vi "Main.vi"(0 "?":bool, 3 "P_max":dbl, 4 "Numbers_of_\nsamples":i32, 5 "V_max":dbl, 6 "V_min":dbl) -> (1 "Progress":u8(slide) scale=0.0..100.0, 2 "I=f(U)":cluster{dbl[], dbl[]}(graph))   [LabVIEW 2020]
doc: "Main VI with state machine.\nMain functions:\n- Ploting graph in real time (Measurment button),\n- Exporting to MS Excel file (Save button),\n- Emergency stop (Stop button),\n- Shutting down application (Exit button)\nInputs:\n- Minimal voltage,\n- Maximum Voltage,\n- Threshold current,\n- Maximum power,\n- Number of measurement samples,\nVisual representation:\n- Graph,\n- Handsome_meater (light on when handsom graph is ploted),\n- Chadomeater (light on when everything is alright),\n- Progressbar,\nExtra features:\n- Playing music during computing,\n- Showing up Cleopatra at the and of measurments,\n- Shuting down with additional sound and picture."
uses:
  <vilib>/sound2/lvsound2.llb/Sound Output Task ID.ctl
  controls/State.ctl
  <vilib>/Analysis/1siggen.llb/Ramp Pattern by Samples.vi
  <vilib>/Utility/error.llb/Error Cluster From Error Code.vi
  <vilib>/ErrorRing/Error Ring.xnode
  <vilib>/Analysis/NI_AALBase.lvlib
panel:
  out "path":path
  out "task ID 2":T1 format="%.0x"
  out "?":picture
  out "2D Picture":picture
  out "task ID":T1 format="%.0x"
  in  "I_max":dbl
  out "Handsom_meter":bool
  out "Chadometer":bool
  in  "?":bool
  in  "?":bool
  in  "?":bool
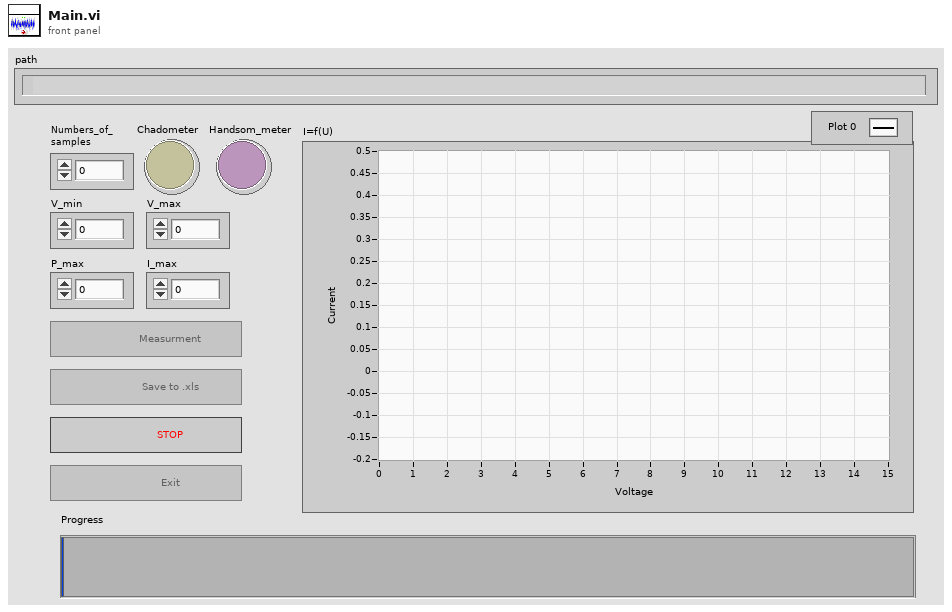
[diagram p1: front panel]
types:
  T1 = typedef "Sound Output Task ID.ctl" = u32
  T2 = typedef "State.ctl" = enum16{"Initialize", "Wait for Event", "Measure", "Save", "Exit"}
  T3 = enum8{"Enabled", "Disabled", "Disabled and Grayed Out"}
  T4 = typedef "imagedata.ctl" = cluster{"image type":i32, "image depth":i32, "image":u8[], "mask":u8[], "colors":u32[], "Rectangle":cluster{"left":i16, "top":i16, "right":i16, "bottom":i16}}
  T5 = typedef "LVBoundsTypeDef.ctl" = cluster{"Width":u32, "Height":u32}
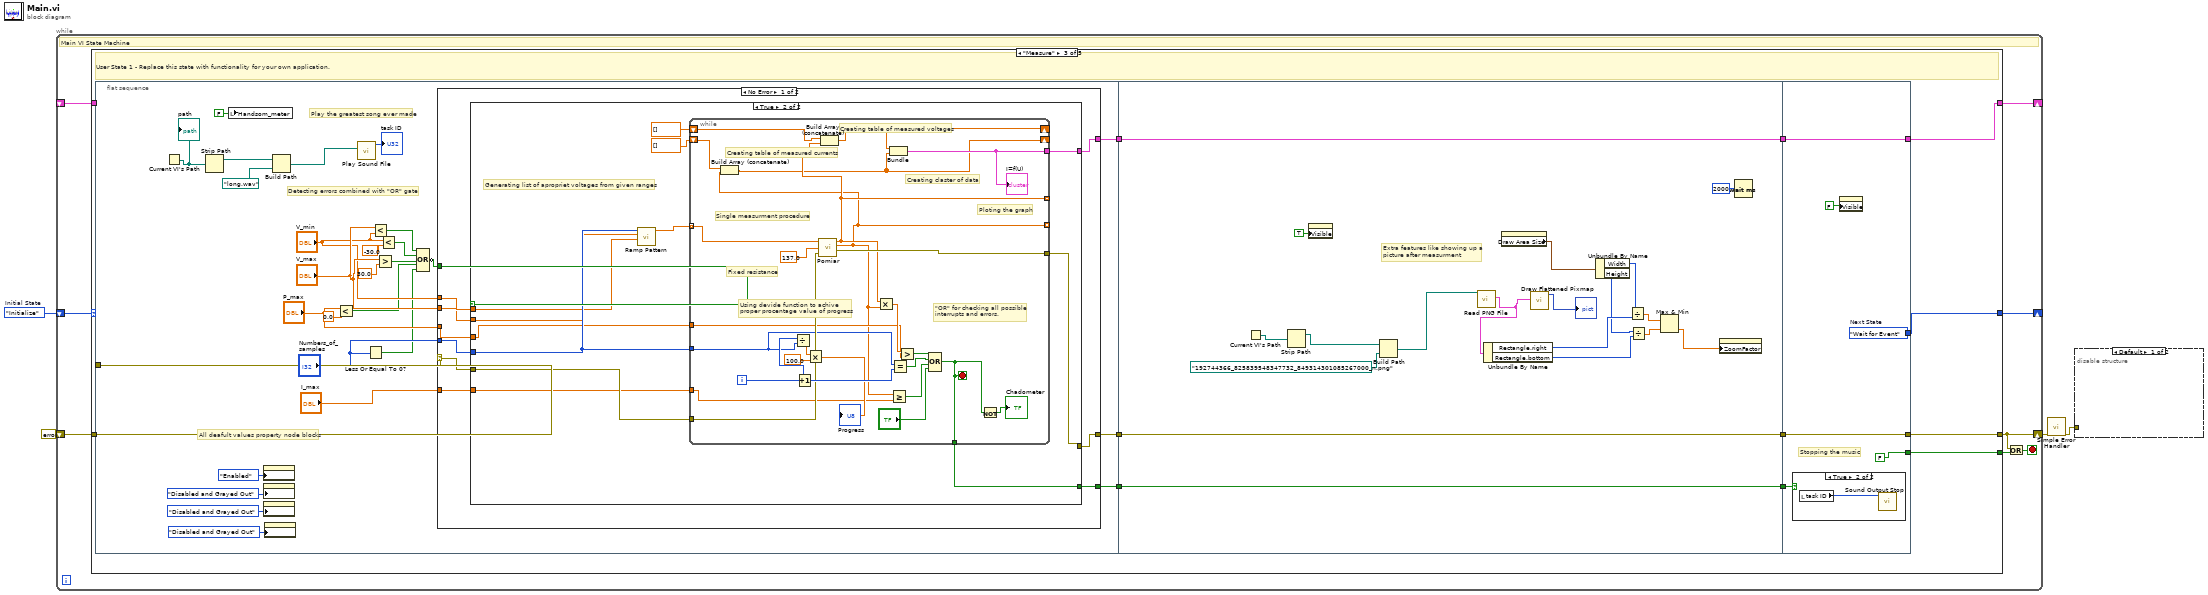
[diagram p0: block diagram]
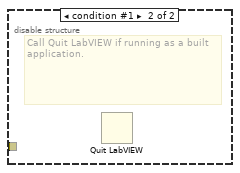
[diagram p2: hidden frame]
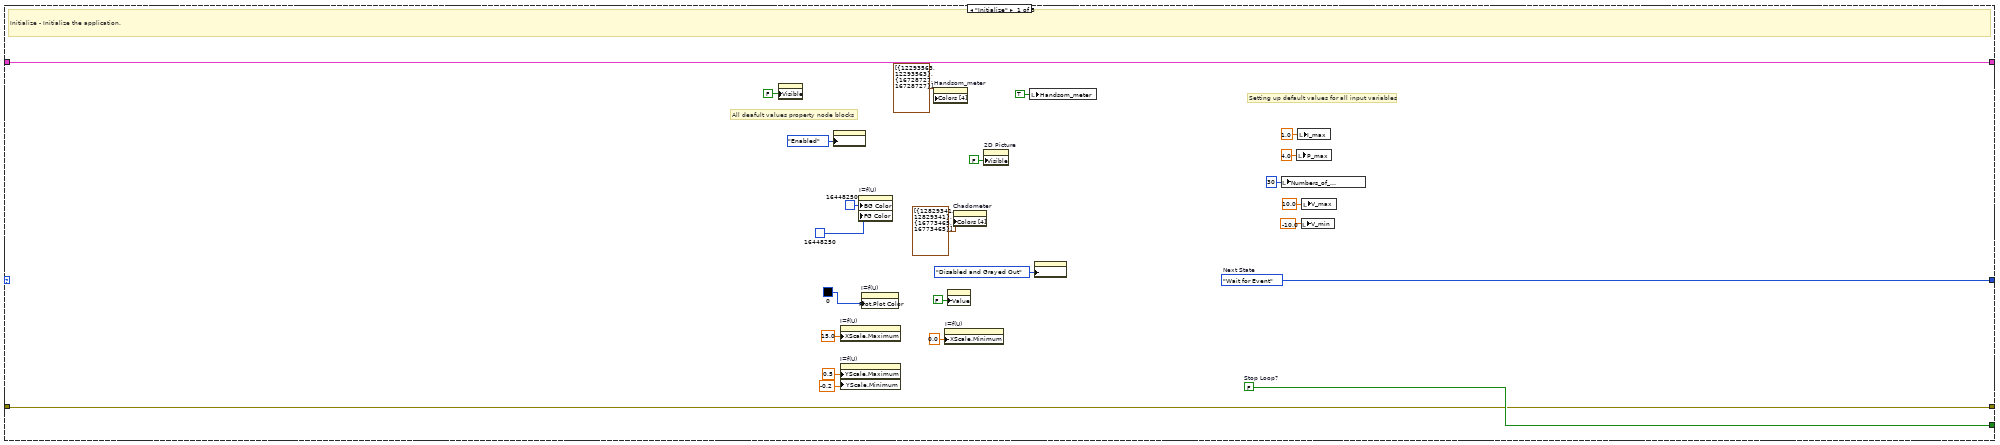
[diagram p3: hidden frame]
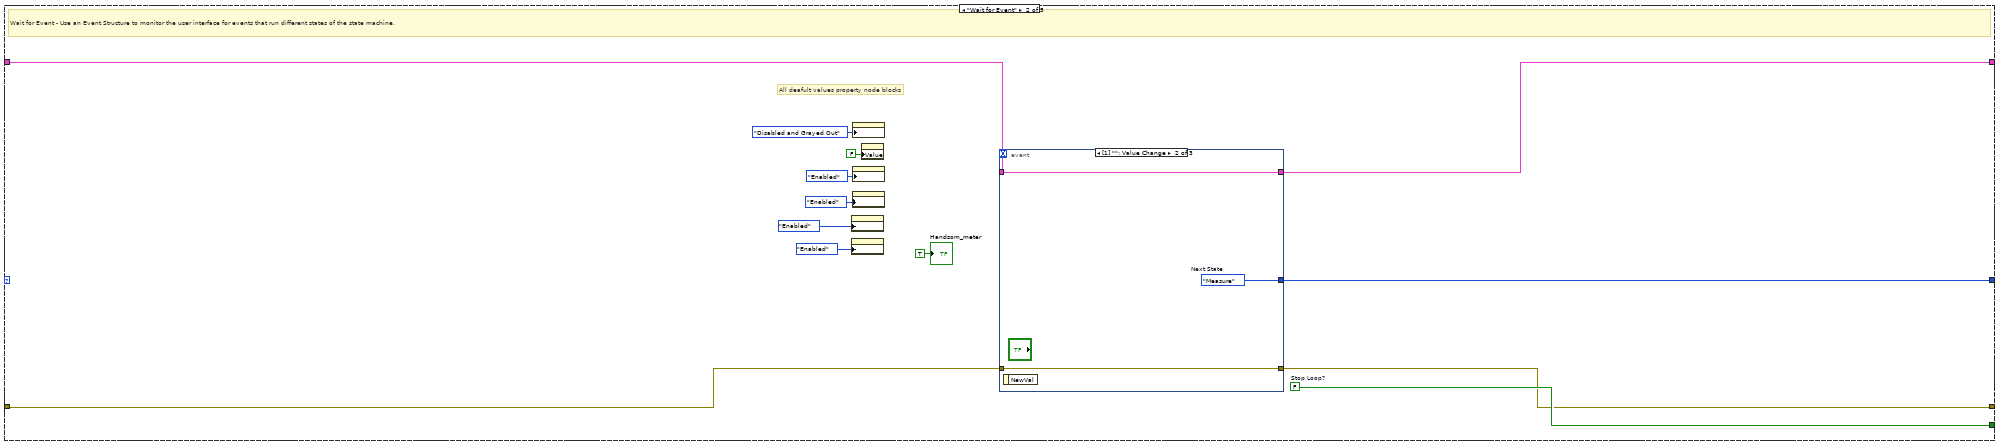
[diagram p4: hidden frame]
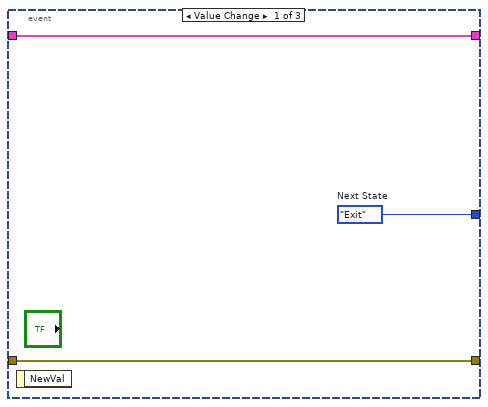
[diagram p5: hidden frame]
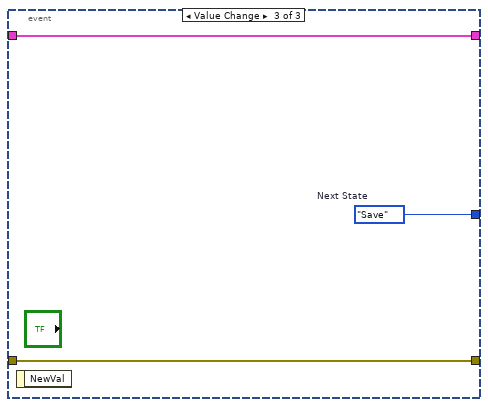
[diagram p6: hidden frame]
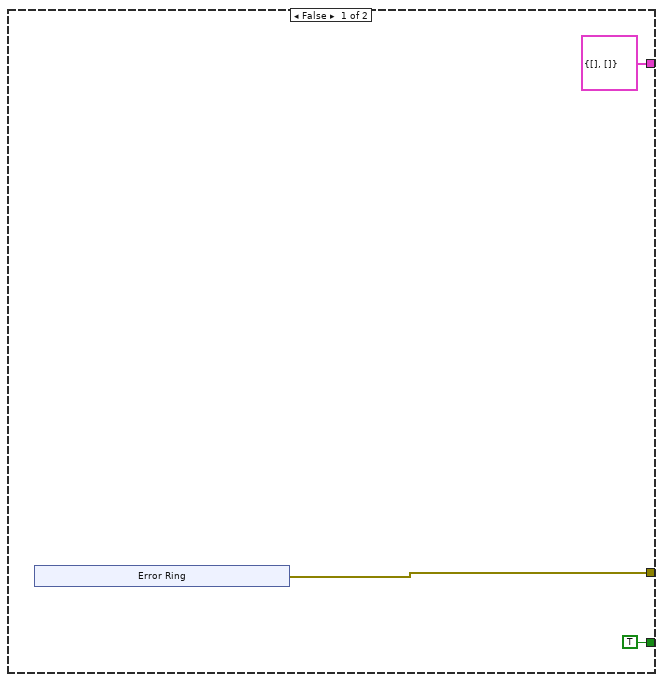
[diagram p7: hidden frame]
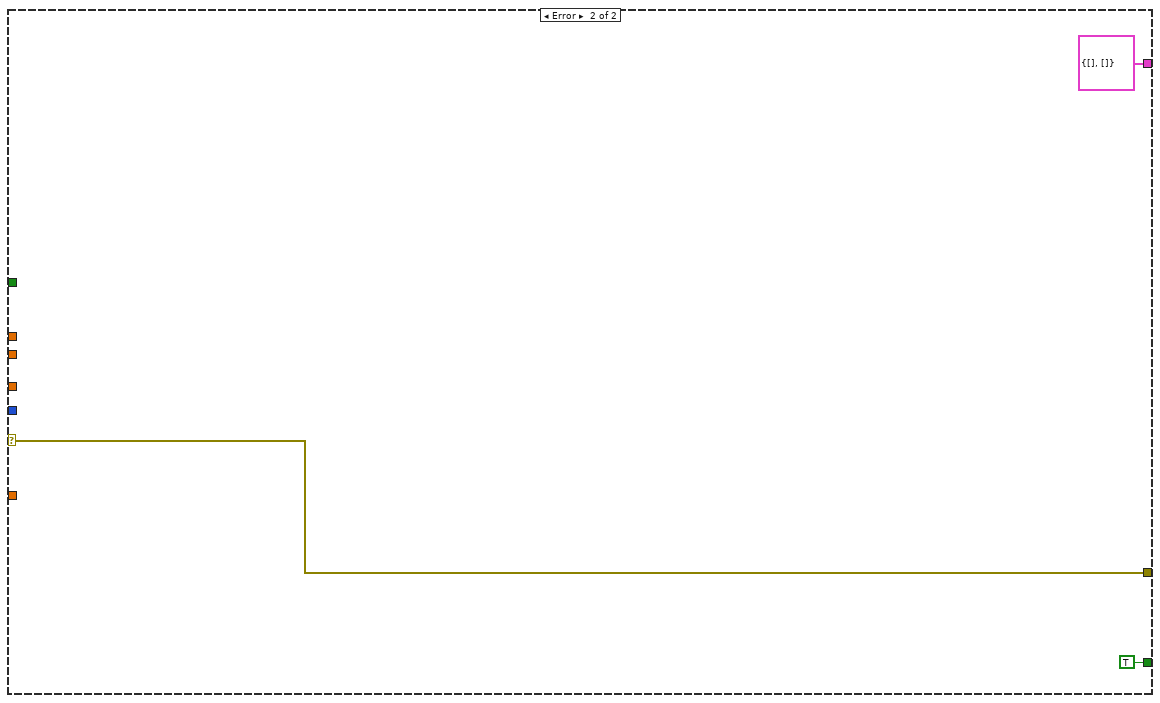
[diagram p8: hidden frame]
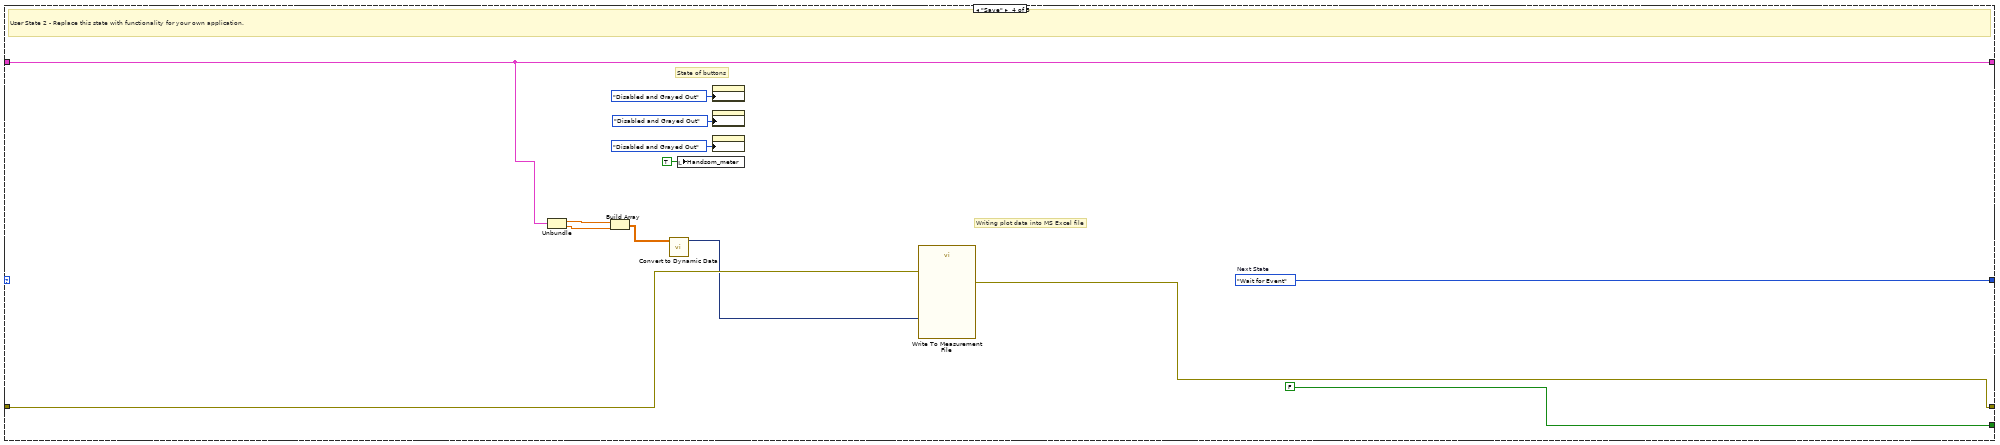
[diagram p10: hidden frame]
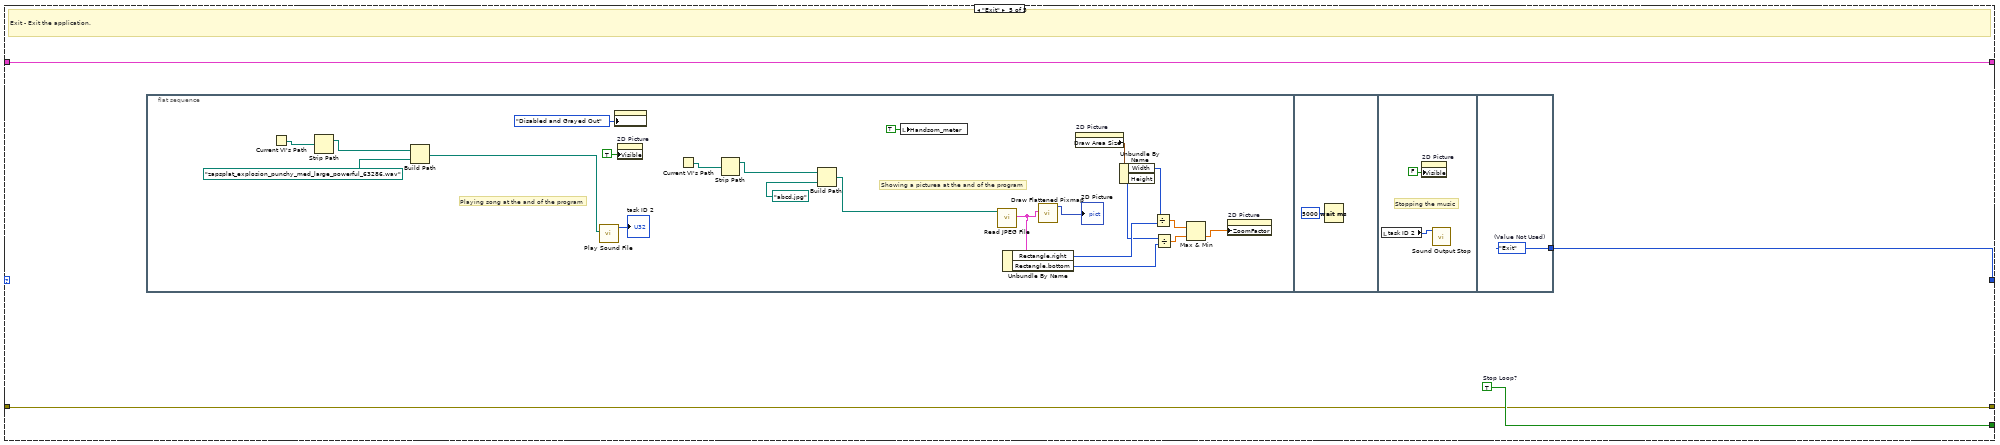
[diagram p11: hidden frame]
diagram:
  w4 = State."Initialize"  # Initial State
  n1 = while {
    shift-right: [w11] -> _
    shift-left: w4 -> [w12]
    shift-right: [w7] -> w2
    shift-left: errorcluster {"status"=FALSE, "code"=0, "source"=""} ("error constant") -> [w10]
    shift-right: [w6] -> _
    shift-left: _ -> [w5]
    stop <- w8 stop-if-true
    # "Main VI State Machine"
    n2 = case shown="\"Measure\"" w12 {
      tunnel: [w36 w49 w61 w195 w196] -> w11
      tunnel: [w35 w48 w62 FALSE ("Stop Loop?") w199] -> w9
      tunnel: w10 -> [w34 w47 w69 w193 w197]
      tunnel: [w34 w46 w68 w192 w197] -> w7
      tunnel: [w29 w44 w67 w189 w198] -> w6
      tunnel: w5 -> [w29 w45 _ w189 w198]
      frame "Initialize" {
        w35 = FALSE  # Stop Loop?
        w36 = State."Wait for Event"  # Next State
        # "Setting up default values for all input variables"
        # "All deafult values property node blocks"
        # "Initialize - Initialize the application."
        n3 = property class="Pict"("Visible"=FALSE) -> ()  [unwired: 2 in, 2 out]
        n4 = property class="Bool"("DisabledEnum"=T3."Enabled" ("Disabled")) -> ()  [unwired: 2 in, 2 out]
        n5 = property on="I=f(U)" class="XYGraph (strict)"("XScale.Maximum"=15.0 ("X Scale.Range:Maximum")) -> ()  [unwired: 2 in, 2 out]
        n6 = property on="I=f(U)" class="XYGraph (strict)"("YScale.Maximum"=0.5 ("Y Scale.Range:Maximum"), "YScale.Minimum"=-0.2 ("Y Scale.Range:Minimum")) -> ()  [unwired: 2 in, 2 out]
        n7 = property on="I=f(U)" class="XYGraph (strict)"("BG Color"=u32 16448250 ("Plot Area:Colors:BG Color"), "FG Color"=u32 16448250 ("Plot Area:Colors:FG Color")) -> ()  [unwired: 2 in, 2 out]
        n8 = property on="I=f(U)" class="XYGraph (strict)"("Plot.Plot Color"=u32 0) -> ()  [unwired: 2 in, 2 out]
        n9 = property on="Handsom_meter" class="Bool (strict)"("Colors [4]"=cluster{u32, u32}[] [{12293563, 12293563}, {16728727, 16728727}]) -> ()  [unwired: 2 in, 2 out]
        n10 = property on="I=f(U)" class="XYGraph (strict)"("XScale.Minimum"=0.0 ("X Scale.Range:Minimum")) -> ()  [unwired: 2 in, 2 out]
        n11 = property class="Bool (strict)"("Value"=FALSE) -> ()  [unwired: 2 in, 2 out]
        n12 = property on="Chadometer" class="Bool (strict)"("Colors [4]"=cluster{u32, u32}[] [{12829341, 12829341}, {16773465, 16773465}]) -> ()  [unwired: 2 in, 2 out]
        n13 = property on="2D Picture" class="Pict"("Visible"=FALSE) -> ()  [unwired: 2 in, 2 out]
        n14 = local write "Handsom_meter"(TRUE ("Handsom_meter")) -> ()
        n15 = property class="Bool (strict)"("DisabledEnum"=T3."Disabled and Grayed Out" ("Disabled")) -> ()  [unwired: 2 in, 2 out]
        n16 = local write "Numbers_of_\nsamples"(30 ("Numbers_of_samples")) -> ()
        n17 = local write "P_max"(4.0 ("P_max")) -> ()
        n18 = local write "I_max"(1.0 ("I_max")) -> ()
        n19 = local write "V_min"(-10.0 ("V_min")) -> ()
        n20 = local write "V_max"(10.0 ("V_max")) -> ()
      }
      frame "Wait for Event" {
        w48 = FALSE  # Stop Loop?
        # "All deafult values property node blocks"
        # "Wait for Event - Use an Event Structure to monitor the user interface for events that run different states of the state machine."
        n21 = property class="Bool"("DisabledEnum"=T3."Enabled" ("Disabled")) -> ()  [unwired: 2 in, 2 out]
        n22 = property class="Bool"("DisabledEnum"=T3."Enabled" ("Disabled")) -> ()  [unwired: 2 in, 2 out]
        n23 = property class="Bool"("DisabledEnum"=T3."Enabled" ("Disabled")) -> ()  [unwired: 2 in, 2 out]
        n24 = property class="Bool (strict)"("DisabledEnum"=T3."Disabled and Grayed Out" ("Disabled")) -> ()  [unwired: 2 in, 2 out]
        n25 = property class="Bool"("DisabledEnum"=T3."Enabled" ("Disabled")) -> ()  [unwired: 2 in, 2 out]
        n26 = property class="Bool (strict)"("Value"=FALSE) -> ()  [unwired: 2 in, 2 out]
        n27 = event shown="[1] \"\": Value Change" {
          selector: _ -> [_ _ _]
          dyn-events: _ -> [_ _ _]
          timeout: _ -> [_ _ _]
          tunnel: [w52 w55 w58] -> w49
          tunnel: w47 -> [w51 w54 w57]
          tunnel: [w51 w54 w57] -> w46
          tunnel: [w50 w53 w56] -> w44
          tunnel: w45 -> [w50 w53 w56]
          event Value Change {
            w52 = State."Exit"  # Next State
            n28 = event-data() -> ()  [unwired: 1 in, 1 out]
          }
          event Value Change {
            w55 = State."Measure"  # Next State
            n29 = event-data() -> ()  [unwired: 1 in, 1 out]
          }
          event Value Change {
            w58 = State."Save"  # Next State
            n30 = event-data() -> ()  [unwired: 1 in, 1 out]
          }
        }
        "Handsom_meter" <- TRUE ("Handsom_meter")
      }
      frame "Measure" {
        # "User State 1 - Replace this state with functionality for your own application."
        n31 = flat-sequence {
          tunnel: w69 -> [w97]
          tunnel: [w82] -> w66
          tunnel: [w81] -> w65
          tunnel: [w74] -> w59
          tunnel: w66 -> [w175]
          tunnel: w65 -> [w174]
          tunnel: [w175] -> w64
          tunnel: [w174] -> w63
          tunnel: [w161] -> w60
          tunnel: w59 -> [w161]
          tunnel: [w180] -> w67
          tunnel: [w181] -> w68
          tunnel: w64 -> [w181]
          tunnel: w63 -> [w180]
          tunnel: [FALSE ("Stop Loop?")] -> w62
          tunnel: [w177] -> w61
          tunnel: w60 -> [w176]
          frame #0 {
            # "Detecting errors combined with \"OR\" gate"
            # "All deafult values property node blocks"
            # "Play the greatest song ever made"
            n32 = Current VI's Path() -> (path=w72:path)
            "path" <- w72
            n33 = Strip Path(path=w72) -> (stripped path=w71:path)  [unwired: 1 out]
            n34 = local write "Handsom_meter"(FALSE ("Handsom_meter")) -> ()
            n35 = property class="Bool (strict)"("DisabledEnum"=T3."Enabled" ("Disabled")) -> ()  [unwired: 2 in, 2 out]
            n36 = property class="Bool"("DisabledEnum"=T3."Disabled and Grayed Out" ("Disabled")) -> ()  [unwired: 2 in, 2 out]
            n37 = property class="Bool"("DisabledEnum"=T3."Disabled and Grayed Out" ("Disabled")) -> ()  [unwired: 2 in, 2 out]
            n38 = property class="Bool"("DisabledEnum"=T3."Disabled and Grayed Out" ("Disabled")) -> ()  [unwired: 2 in, 2 out]
            n39 = Build Path(base path=w71, name or relative path=path "long.wav") -> (appended path=w70:path)
            n40 = Less?(x="P_max", y=0.0) -> (x < y?=w86:bool)
            n41 = call <vilib>:"Play Sound File.vi"("path"=w70) -> ("task ID"=→"task ID":T1)  [unwired: 9 in, 1 out]
            n42 = Less Or Equal To 0?(x="Numbers_of_\nsamples") -> (x <= 0?=w85:bool)
            n43 = Less?(x="V_max", y="V_min") -> (x < y?=w89:bool)
            n44 = Greater?(x="V_max", y=30.0) -> (0:w87:bool)
            n45 = Less?(x="V_min", y=-30.0) -> (x < y?=w88:bool)
            n46 = Compound Arithmetic op=OR(w89, w88, w87, w86, w85) -> (invert w83:bool)
            n47 = case shown="No Error" w97 {
              selector: w97 -> [w103 w156]
              tunnel: "V_min" -> [w107 _]
              tunnel: "V_max" -> [w106 _]
              tunnel: "P_max" -> [w105 _]
              tunnel: "Numbers_of_\nsamples" -> [w104 _]
              tunnel: w83 -> [w102 _]
              tunnel: [w101 w156] -> w82
              tunnel: [w100 cluster{dbl[], dbl[]} {[], []}] -> w81
              tunnel: "I_max" -> [w99 _]
              tunnel: [w98 TRUE] -> w74
              frame No Error {
                n48 = case shown="True" w102 {
                  tunnel: w107 -> [_ w121]
                  tunnel: w106 -> [_ w122]
                  tunnel: w105 -> [_ w123]
                  tunnel: w104 -> [_ w124]
                  tunnel: w103 -> [_ w126]
                  tunnel: [w110 w125] -> w101
                  tunnel: [cluster{dbl[], dbl[]} {[], []} w120] -> w100
                  tunnel: w99 -> [_ w117]
                  tunnel: [TRUE w116] -> w98
                  frame False {
                    n49 = xnode "Error Ring"() -> ("error out"=w110:errorcluster)
                  }
                  frame True {
                    # "Generating list of apropriet voltages from given ranges"
                    n50 = call-poly <vilib>:"Ramp Pattern.vi"("start"=w121, "end"=w122, "samples"=w124) -> ("Ramp Pattern"=w127:dbl[])  [unwired: 7 in, 1 out]
                    n51 = while {
                      tunnel: w127 -> [w153] mode=indexing
                      tunnel: [w137] -> _ mode=indexing
                      tunnel: [w132] -> _ mode=indexing
                      tunnel: [w147] -> w125
                      tunnel: w126 -> [w143]
                      tunnel: w124 -> [w142]
                      tunnel: w123 -> [w141]
                      shift-right: [w128] -> _
                      shift-left: dbl[] [] -> [w138]
                      shift-right: [w129] -> _
                      shift-left: dbl[] [] -> [w136]
                      tunnel: [w139] -> w120
                      tunnel: [w135] -> w116
                      tunnel: w117 -> [w131]
                      i -> [w150]
                      stop <- w135 stop-if-true
                      # "\"OR\" for checking all possible\ninterrupts and errors."
                      # "Using devide function to achive \nproper procentage value of progress"
                      # "Ploting the graph"
                      # "Creating claster of data"
                      # "Creating table of measured currents"
                      # "Creating table of measured voltages"
                      # "Fixed resistance"
                      # "Single measurment procedure"
                      n52 = Increment(x=w150) -> (x+1=w146:i32)
                      n53 = Divide(x=w146, y=w142) -> (x/y=w145:dbl)
                      n54 = Multiply(x=w145, y=100.0) -> (x*y=→"Progress":dbl)
                      n55 = call "Pomiar.vi"("Voltage"=w153, "Resistance"=137.0, "error in (no error)"=w143) -> ("Voltage output"=w137:dbl, "Current output"=w132:dbl, "error out"=w147:errorcluster)  [unwired: 1 in]
                      n56 = Build Array (concatenate)(w136, w132) -> (w129:dbl[])
                      n57 = Build Array (concatenate)(w138, w137) -> (w128:dbl[])
                      n58 = Multiply(x=w137, y=w132) -> (x*y=w152:dbl)
                      n59 = Bundle(w128, w129) -> (w139:cluster{dbl[], dbl[]})  [unwired: 1 in]
                      "I=f(U)" <- w139
                      n60 = Greater Or Equal?(x=w132, y=w131) -> (x >= y?=w133:bool)
                      n61 = Equal?(x=w142, y=w146) -> (x = y?=w148:bool)
                      n62 = Greater?(x=w152, y=w141) -> (0:w149:bool)
                      n63 = Compound Arithmetic op=OR(w149, w148, w133, "?") -> (w135:bool)
                      n64 = Not(x=w135) -> (.not. x?=→"Chadometer":bool)
                    }
                  }
                }
              }
              frame Error {
              }
            }
          }
          frame #1 {
            # "Extra features like showing up a \npicture after measurment"
            n65 = Current VI's Path() -> (path=w159:path)
            n66 = Strip Path(path=w159) -> (stripped path=w158:path)  [unwired: 1 out]
            n67 = property class="Pict"("Visible"=TRUE) -> ()  [unwired: 2 in, 2 out]
            n68 = Build Path(base path=w158, name or relative path=path "192744366_825839548347732_849314301085267000_n.png") -> (appended path=w157:path)
            n69 = call <vilib>:"Read PNG File.vi"("path to PNG file"=w157) -> ("image data"=w162:T4)  [unwired: 8 in, 2 out]
            n70 = Unbundle By Name(w162) -> ("Rectangle.right"=w173:i16, "Rectangle.bottom"=w172:i16)
            n71 = property class="Pict"() -> ("Draw Area Size"=w168:T5)  [unwired: 2 in, 2 out]
            n72 = call <vilib>:"Draw Flattened Pixmap.vi"("image data"=w162) -> ("new picture"=→"?":picture)  [unwired: 8 in]
            n73 = Unbundle By Name(w168) -> ("Width"=w166:u32, "Height"=w167:u32)
            n74 = Divide(x=w166, y=w173) -> (x/y=w171:dbl)
            n75 = Divide(x=w167, y=w172) -> (x/y=w170:dbl)
            n76 = Max & Min(x=w171, y=w170) -> (min(x,y)=w165:dbl)  [unwired: 1 out]
            n77 = property class="Pict"("ZoomFactor"=w165) -> ()  [unwired: 2 in, 2 out]
            n78 = Wait (ms)(milliseconds to wait=u32 2000) -> ()  [unwired: 1 out]
          }
          frame #2 {
            w177 = State."Wait for Event"  # Next State
            # "Stopping the music"
            n79 = case shown="True" w176 {
              frame False {
              }
              frame True {
                n80 = local read "task ID"() -> (w182:T1)
                n81 = call <vilib>:"Sound Output Stop.vi"("task ID"=w182) -> ()  [unwired: 9 in, 2 out]
              }
            }
            n82 = property class="Pict"("Visible"=FALSE) -> ()  [unwired: 2 in, 2 out]
          }
        }
      }
      frame "Save" {
        w195 = State."Wait for Event"  # Next State
        # "State of buttons"
        # "Writing plot data into MS Excel file"
        # "User State 2 - Replace this state with functionality for your own application."
        n83 = Unbundle(w189) -> (w188:dbl[], w187:dbl[])
        n84 = Build Array(w188, w187) -> (w191:dbl[][])
        n85 = call "Convert to Dynamic Data"("2D Array"=w191) -> ("Dynamic Data Type"=w190:dynamicdata)  [unwired: 3 in]
        n86 = local write "Handsom_meter"(TRUE ("Handsom_meter")) -> ()
        n87 = property class="Bool (strict)"("DisabledEnum"=T3."Disabled and Grayed Out" ("Disabled")) -> ()  [unwired: 2 in, 2 out]
        n88 = property class="Bool"("DisabledEnum"=T3."Disabled and Grayed Out" ("Disabled")) -> ()  [unwired: 2 in, 2 out]
        n89 = property class="Bool"("DisabledEnum"=T3."Disabled and Grayed Out" ("Disabled")) -> ()  [unwired: 2 in, 2 out]
        n90 = call "Write To Measurement File"("Signals"=w190, "error in (no error)"=w193) -> ("error out"=w192:errorcluster)  [unwired: 15 in, 2 out]
      }
      frame "Exit" {
        w199 = TRUE  # Stop Loop?
        # "Exit - Exit the application."
        n91 = flat-sequence {
          tunnel: [w225] -> w196
          frame #0 {
            # "Showing a picturea at the and of the program"
            # "Playing song at the and of the program"
            n92 = Current VI's Path() -> (path=w207:path)
            n93 = Strip Path(path=w207) -> (stripped path=w206:path)  [unwired: 1 out]
            n94 = Build Path(base path=w206, name or relative path=path "zapsplat_explosion_punchy_med_large_powerful_63286.wav") -> (appended path=w204:path)
            n95 = call <vilib>:"Play Sound File.vi"("path"=w204) -> ("task ID"=→"task ID 2":T1)  [unwired: 9 in, 1 out]
            n96 = property class="Bool (strict)"("DisabledEnum"=T3."Disabled and Grayed Out" ("Disabled")) -> ()  [unwired: 2 in, 2 out]
            n97 = property on="2D Picture" class="Pict"("Visible"=TRUE) -> ()  [unwired: 2 in, 2 out]
            n98 = Current VI's Path() -> (path=w202:path)
            n99 = Strip Path(path=w202) -> (stripped path=w201:path)  [unwired: 1 out]
            n100 = Build Path(base path=w201, name or relative path=path "abcd.jpg") -> (appended path=w200:path)
            n101 = local write "Handsom_meter"(TRUE ("Handsom_meter")) -> ()
            n102 = call <vilib>:"Read JPEG File.vi"("path to JPEG file"=w200) -> ("image data"=w219:T4)  [unwired: 8 in, 2 out]
            n103 = Unbundle By Name(w219) -> ("Rectangle.right"=w218:i16, "Rectangle.bottom"=w217:i16)
            n104 = call <vilib>:"Draw Flattened Pixmap.vi"("image data"=w219) -> ("new picture"=→"2D Picture":picture)  [unwired: 8 in]
            n105 = property on="2D Picture" class="Pict"() -> ("Draw Area Size"=w213:T5)  [unwired: 2 in, 2 out]
            n106 = Unbundle By Name(w213) -> ("Width"=w211:u32, "Height"=w212:u32)
            n107 = Divide(x=w211, y=w218) -> (x/y=w216:dbl)
            n108 = Divide(x=w212, y=w217) -> (x/y=w215:dbl)
            n109 = Max & Min(x=w216, y=w215) -> (min(x,y)=w214:dbl)  [unwired: 1 out]
            n110 = property on="2D Picture" class="Pict"("ZoomFactor"=w214) -> ()  [unwired: 2 in, 2 out]
          }
          frame #1 {
            n111 = Wait (ms)(milliseconds to wait=u32 5000) -> ()  [unwired: 1 out]
          }
          frame #2 {
            # "Stopping the music"
            n112 = local read "task ID 2"() -> (w223:T1)
            n113 = property on="2D Picture" class="Pict"("Visible"=FALSE) -> ()  [unwired: 2 in, 2 out]
            n114 = call <vilib>:"Sound Output Stop.vi"("task ID"=w223) -> ()  [unwired: 9 in, 2 out]
          }
          frame #3 {
            w225 = State."Exit"  # (Value Not Used)
          }
        }
      }
    }
    n115 = Or(x=w7, y=w9) -> (x .or. y?=w8:bool)
  }
  n116 = call <vilib>:"Simple Error Handler.vi"("error in (no error)"=w2) -> ("error out"=w1:errorcluster)  [unwired: 4 in, 4 out]
  n117 = disable-structure shown="Default" {
    disable-tunnel: w1 -> [_ _]
    frame condition #0 (active) {
    }
    frame condition #1 {
      # "Call Quit LabVIEW if running as a built application."
      n118 = Quit LabVIEW() -> ()  [unwired: 1 in]
    }
  }
